vi "3D Model of Solar System.vi"() -> ()   [LabVIEW 2016]
doc: "This example demonstrates some fundamental concepts for the 3D picture. Concepts covered include object creation, texturing, object movement, and object hierarchy."
uses:
  <vilib>/Utility/miscctls.llb/LVRectTypeDef.ctl
  <vilib>/picture/3D Picture Control/Object/Create Object (drawable).vi
  <vilib>/picture/3D Picture Control/Helpers/Apply Texture (no reference).vi
  <vilib>/picture/3D Picture Control/Object/Create Object (name).vi
  <vilib>/picture/3D Picture Control/Object/Add Object (reference).vi
  <vilib>/picture/3D Picture Control/NI_3D Picture Control.lvlib
panel:
  in  "Rendering Destination":enum16{"Scene Window", "Scene Display"}(ring)=enum."Scene Display"
  in  "Camera Controller":enum16{"None", "Spherical", "Flying"}(ring)=enum."Spherical"
  out "Scene Display":refnum<vi>(3d-picture)
  in  "Stop":bool
  # "Overview: This example demonstrates some fundamental concepts for the 3D Picture by animating an image of the solar system.\nRequirements: LabVIEW Full Development System\nInstructions: \n1. Choose the Rendering Destination. If you choose Scene Window, a new window will show the rendering of the solar system. If you choose Scene Display, the picture will be shown in the Scene Display indicator on this front panel. \n2. Run the VI to see the animation of the solar system. \n3. Click Stop to stop the VI."
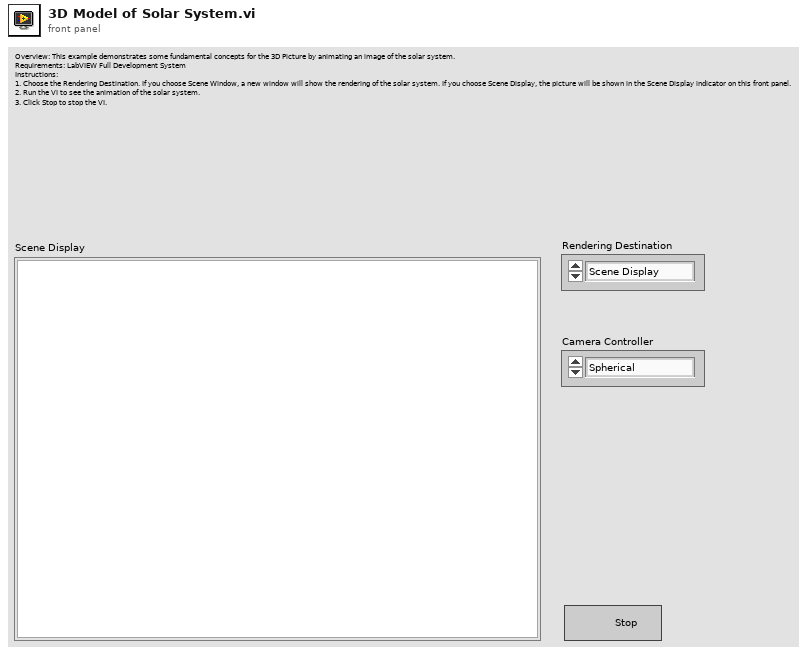
[diagram p1: front panel]
types:
  T1 = enum16{"As a Decal", "With Modulation", "With Blending", "As a replacement"}
  T2 = enum16{"No Filtration", "Linear Filtration", "Simple Mipmap Filtration", "Bilinear Filtration", "Trilinear Filtration"}
  T3 = typedef "imagedata.ctl" = cluster{"image type":i32, "image depth":i32, "image":u8[], "mask":u8[], "colors":u32[], "Rectangle":cluster{"left":i16, "top":i16, "right":i16, "bottom":i16}}
  T4 = enum16{"Open", "Minimized", "Maximized", "Hidden"}
  T5 = typedef "LVRectTypeDef.ctl" = cluster{"Left":i16, "Top":i16, "Right":i16, "Bottom":i16}
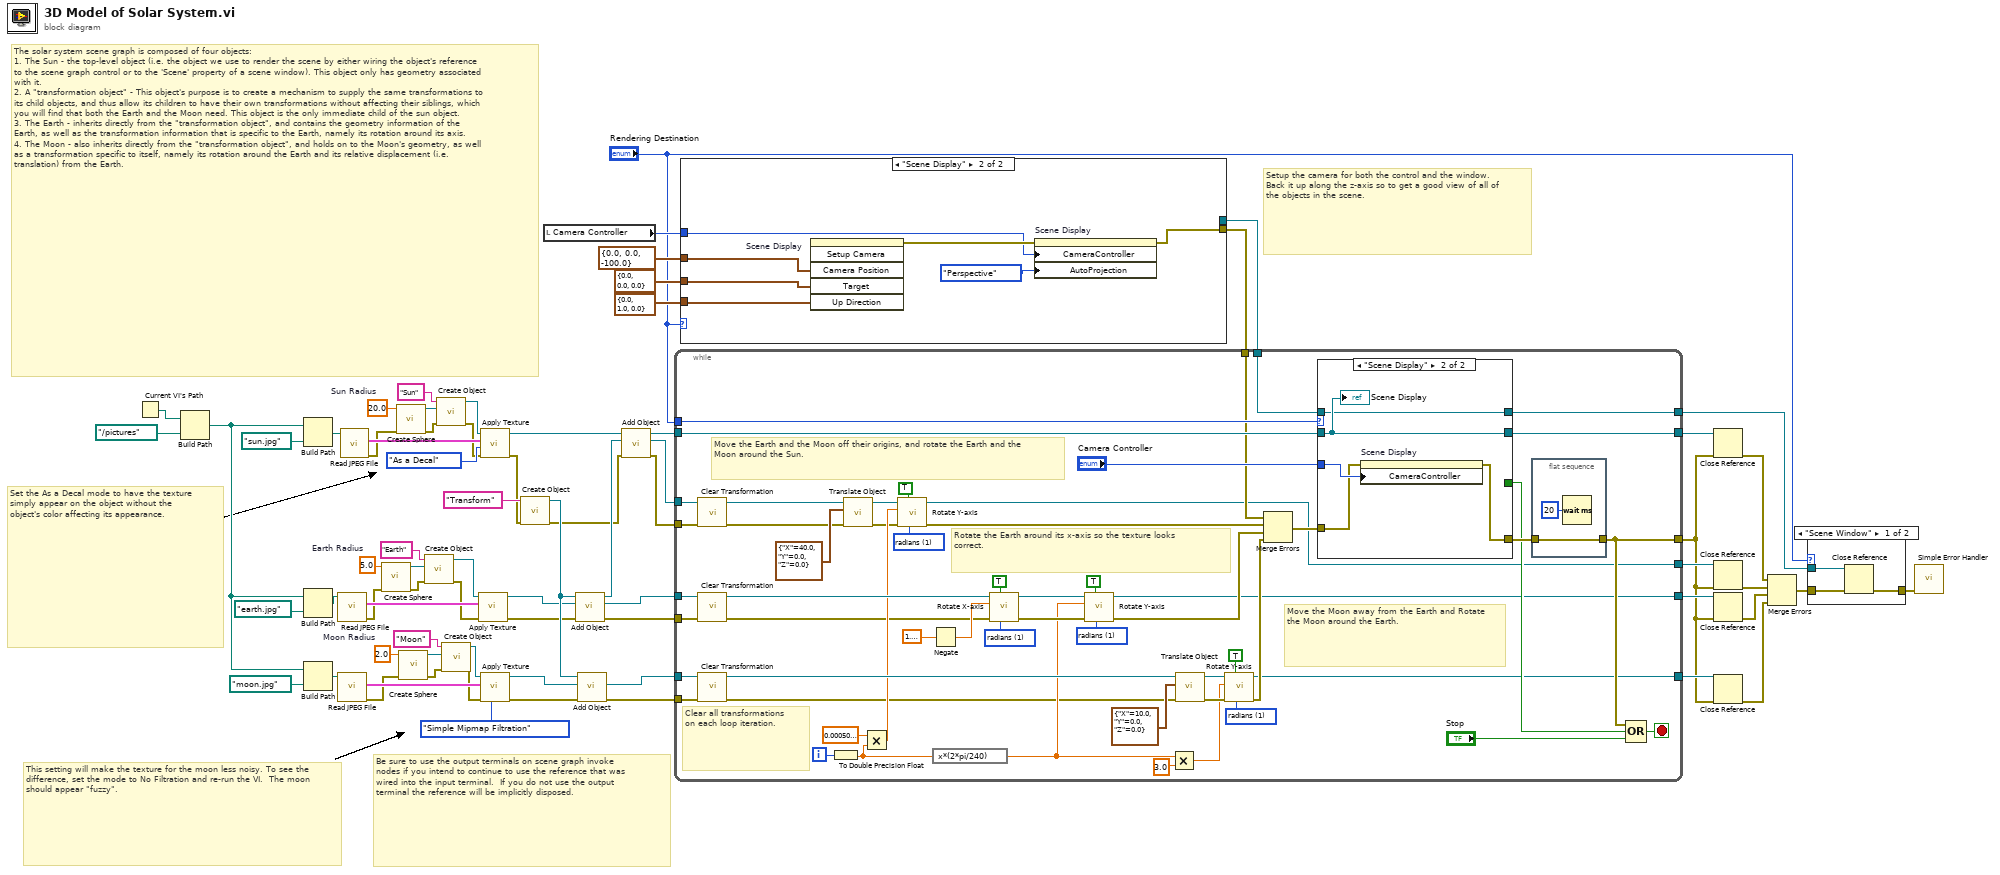
[diagram p0: block diagram]
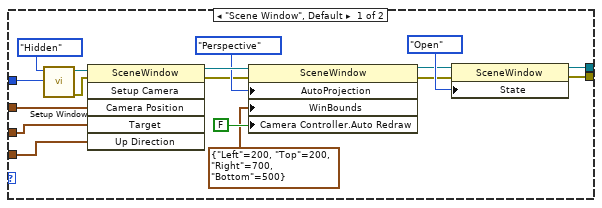
[diagram p3: hidden frame]
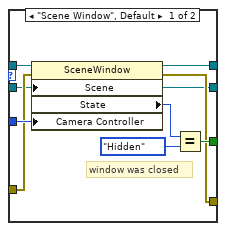
[diagram p4: hidden frame]
diagram:
  w68 = sgl 2.0  # Moon Radius
  w69 = sgl 5.0  # Earth Radius
  w70 = sgl 20.0  # Sun Radius
  # "Set the As a Decal mode to have the texture simply appear on the object without the object's color affecting its appearance."
  # "This setting will make the texture for the moon less noisy. To see the difference, set the mode to No Filtration and re-run the VI.  The moon should appear \"fuzzy\"."
  # "Be sure to use the output terminals on scene graph invoke nodes if you intend to continue to use the reference that was wired into the input terminal.  If you do not use the output terminal the reference will be implicitly disposed."
  # "Setup the camera for both the control and the window.  Back it up along the z-axis so to get a good view of all of the objects in the scene."
  # "The solar system scene graph is composed of four objects:\n1. The Sun - the top-level object (i.e. the object we use to render the scene by either wiring the object's reference to the scene graph control or to the 'Scene' property of a scene window). This object only has geometry associated with it.\n2. A \"transformation object\" - This object's purpose is to create a mechanism to supply the same transformations to its child objects, and thus allow its children to have their own transformations without affecting their siblings, which you will find that both the Earth and the Moon need. This object is the only immediate child of the sun object.\n3. The Earth - inherits directly from the \"transformation object\", and contains the geometry information of the Earth, as well as the transformation information that is specific to the Earth, namely its rotation around its axis.\n4. The Moon - also inherits directly from the \"transformation object\", and holds on to the Moon's geometry, as well as a transformation specific to itself, namely its rotation around the Earth and its relative displacement (i.e. translation) from the Earth."
  n1 = Current VI's Path() -> (path=w14:path)
  n2 = Build Path(base path=w14, name or relative path=path "../pictures" ("path")) -> (appended path=w17:path)
  n3 = Build Path(base path=w17, name or relative path=path "sun.jpg" ("Name")) -> (appended path=w66:path)
  n4 = Build Path(base path=w17, name or relative path=path "earth.jpg" ("Name")) -> (appended path=w64:path)
  n5 = Build Path(base path=w17, name or relative path=path "moon.jpg" ("Name")) -> (appended path=w62:path)
  n6 = call <vilib>:"Read JPEG File.vi"("path to JPEG file"=w64) -> ("error out"=w23:errorcluster, "image data"=w44:T3)  [unwired: 1 in, 8 out]
  n7 = call <vilib>:"Read JPEG File.vi"("path to JPEG file"=w62) -> ("error out"=w24:errorcluster, "image data"=w58:T3)  [unwired: 1 in, 8 out]
  n8 = call <vilib>:"Read JPEG File.vi"("path to JPEG file"=w66) -> ("error out"=w22:errorcluster, "image data"=w52:T3)  [unwired: 1 in, 8 out]
  n9 = call <vilib>:"Create Sphere.vi"("error in (no error)"=w23, "Radius"=w69) -> ("error out"=w26:errorcluster, "New Sphere Refnum"=w55:refnum<vi>)  [unwired: 1 in, 7 out]
  n10 = call <vilib>:"Create Sphere.vi"("error in (no error)"=w22, "Radius"=w70) -> ("error out"=w21:errorcluster, "New Sphere Refnum"=w42:refnum<vi>)  [unwired: 1 in, 7 out]
  n11 = call <vilib>:"Create Sphere.vi"("error in (no error)"=w24, "Radius"=w68) -> ("error out"=w28:errorcluster, "New Sphere Refnum"=w60:refnum<vi>)  [unwired: 1 in, 7 out]
  n12 = call-poly <vilib>:"Create Object.vi"("error in (no error)"=w26, "Geometry"=w55, "Name"="Earth") -> ("error out"=w25:errorcluster, "Scene:New Object"=w45:refnum<vi>)  [unwired: 7 in]
  n13 = call-poly <vilib>:"Create Object.vi"("error in (no error)"=w21, "Geometry"=w42, "Name"="Sun") -> ("error out"=w20:errorcluster, "Scene:New Object"=w53:refnum<vi>)  [unwired: 7 in]
  n14 = call-poly <vilib>:"Create Object.vi"("error in (no error)"=w28, "Geometry"=w60, "Name"="Moon") -> ("error out"=w27:errorcluster, "Scene:New Object"=w59:refnum<vi>)  [unwired: 7 in]
  n15 = call-poly <vilib>:"Apply Texture.vi"("error in (no error)"=w25, "Image Data"=w44, "Scene Object In"=w45) -> ("error out"=w34:errorcluster, "Scene Object Out"=w43:refnum<vi>)  [unwired: 7 in]
  n16 = call-poly <vilib>:"Apply Texture.vi"("error in (no error)"=w20, "Apply Mode"=T1."As a Decal", "Image Data"=w52, "Scene Object In"=w53) -> ("error out"=w19:errorcluster, "Scene Object Out"=w51:refnum<vi>)  [unwired: 6 in]
  n17 = call-poly <vilib>:"Apply Texture.vi"("Filter Mode"=T2."Simple Mipmap Filtration", "error in (no error)"=w27, "Image Data"=w58, "Scene Object In"=w59) -> ("error out"=w33:errorcluster, "Scene Object Out"=w57:refnum<vi>)  [unwired: 6 in]
  n18 = call-poly <vilib>:"Create Object.vi"("error in (no error)"=w19, "Name"="Transform") -> ("error out"=w32:errorcluster, "Scene:New Object"=w47:refnum<vi>)  [unwired: 8 in]
  n19 = local read "Camera Controller"() -> (w40:enum16{"None", "Spherical", "Flying"})
  n20 = call-poly <vilib>:"Add Object.vi"("error in (no error)"=w34, "New Object In"=w43, "Scene Object In"=w47) -> ("error out"=w30:errorcluster, "New Object Out"=w48:refnum<vi>, "Scene Object Out"=w46:refnum<vi>)  [unwired: 6 in]
  n21 = call-poly <vilib>:"Add Object.vi"("error in (no error)"=w33, "New Object In"=w57, "Scene Object In"=w47) -> ("error out"=w29:errorcluster, "New Object Out"=w18:refnum<vi>)  [unwired: 6 in, 1 out]
  n22 = call-poly <vilib>:"Add Object.vi"("error in (no error)"=w32, "New Object In"=w46, "Scene Object In"=w51) -> ("error out"=w31:errorcluster, "New Object Out"=w50:refnum<vi>, "Scene Object Out"=w49:refnum<vi>)  [unwired: 6 in]
  n23 = case shown="\"Scene Display\"" "Rendering Destination" {
    tunnel: w40 -> [w79 w93]
    tunnel: cluster{"X":sgl, "Y":sgl, "Z":sgl} {"X"=0.0, "Y"=0.0, "Z"=-100.0} ("Camera Position") -> [w81 w92]
    tunnel: cluster{"X":sgl, "Y":sgl, "Z":sgl} {"X"=0.0, "Y"=0.0, "Z"=0.0} ("Target") -> [w82 w91]
    tunnel: cluster{"X":sgl, "Y":sgl, "Z":sgl} {"X"=0.0, "Y"=1.0, "Z"=0.0} ("Up Direction") -> [w83 w90]
    tunnel: [w76 _] -> w36
    tunnel: [w72 w89] -> w15
    frame "Scene Window", Default {
      n24 = call <vilib>:"Setup Window.vi"("Camera Controller"=w79, "Window State"=T4."Hidden") -> ("error out"=w75:errorcluster, "New Window Refnum"=w85:refnum<vi>)  [unwired: 1 in, 7 out]
      n25 = invoke class="SceneWindow" method="Setup Camera"(reference=w85, error in=w75, "Camera Position"=w81, "Target"=w82, "Up Direction"=w83) -> (reference out=w84:refnum<vi>, error out=w74:errorcluster)  [unwired: 1 in, 4 out]
      n26 = property class="SceneWindow"(reference=w84, error in=w74, "AutoProjection"=enum16{"None", "Perspective", "Orthographic"}."Perspective" ("Automatic Projection Mode"), "WinBounds"=T5 {"Left"=200, "Top"=200, "Right"=700, "Bottom"=500} ("Window Bounds"), "Camera Controller.Auto Redraw"=FALSE ("Camera Controller:Auto Redraw")) -> (reference out=w77:refnum<vi>, error out=w73:errorcluster)
      n27 = property class="SceneWindow"(reference=w77, error in=w73, "State"=T4."Open" ("Window State")) -> (reference out=w76:refnum<vi>, error out=w72:errorcluster)
    }
    frame "Scene Display" {
      n28 = invoke on="Scene Display" class="SceneGraphDisp (strict)" method="Setup Camera"("Camera Position"=w92, "Target"=w91, "Up Direction"=w90) -> (error out=w94:errorcluster)  [unwired: 3 in, 5 out]
      n29 = property on="Scene Display" class="SceneGraphDisp (strict)"(error in=w94, "CameraController"=w93, "AutoProjection"=enum16{"None", "Perspective", "Orthographic"}."Perspective" ("Auto Projection Mode")) -> (error out=w89:errorcluster)  [unwired: 1 in, 1 out]
    }
  }
  n30 = while {
    tunnel: w36 -> [w149]
    tunnel: w49 -> [w148]
    tunnel: w50 -> [w147]
    tunnel: w48 -> [w146]
    tunnel: w18 -> [w145]
    tunnel: "Rendering Destination" -> [w144]
    tunnel: w31 -> [w115]
    tunnel: w30 -> [w113]
    tunnel: w29 -> [w112]
    tunnel: [w110] -> w4
    tunnel: w15 -> [w103]
    tunnel: [w100] -> w13
    tunnel: [w99] -> w11
    tunnel: [w98] -> w12
    tunnel: [w97] -> w10
    tunnel: [w96] -> w5
    i -> [w151]
    stop <- w111 stop-if-true
    w124 = u16 1 items=["degree", "radians"] ("angle unit")
    w125 = u16 1 items=["degree", "radians"] ("angle unit")
    w126 = u16 1 items=["degree", "radians"] ("angle unit")
    w127 = u16 1 items=["degree", "radians"] ("angle unit")
    # "Move the Moon away from the Earth and Rotate the Moon around the Earth."
    # "Rotate the Earth around its x-axis so the texture looks correct."
    # "Move the Earth and the Moon off their origins, and rotate the Earth and the Moon around the Sun."
    # "Clear all transformations on each loop iteration."
    n31 = call <vilib>:"Clear Transformation.vi"("error in (no error)"=w115, "Object Refnum In"=w147) -> ("error out"=w114:errorcluster, "Object Refnum Out"=w143:refnum<vi>)  [unwired: 8 out]
    n32 = call <vilib>:"Clear Transformation.vi"("error in (no error)"=w113, "Object Refnum In"=w146) -> ("error out"=w109:errorcluster, "Object Refnum Out"=w142:refnum<vi>)  [unwired: 8 out]
    n33 = call <vilib>:"Clear Transformation.vi"("error in (no error)"=w112, "Object Refnum In"=w145) -> ("error out"=w108:errorcluster, "Object Refnum Out"=w141:refnum<vi>)  [unwired: 8 out]
    n34 = To Double Precision Float(number=w151) -> (double precision float=w150:dbl)
    n35 = call <vilib>:"Translate Object.vi"("error in (no error)"=w114, "Translation"=cluster{"X":sgl, "Y":sgl, "Z":sgl} {"X"=40.0, "Y"=0.0, "Z"=0.0}, "Scene.Object In"=w143) -> ("error out"=w135:errorcluster, "Scene.Object Out"=w136:refnum<vi>)  [unwired: 7 out]
    n36 = Multiply(x=sgl 0.0005 ("Angle"), y=w150) -> (x*y=w139:dbl)
    n37 = call <vilib>:"Rotate Y-axis.vi"("angle unit"=w124, "Relative?"=TRUE, "error in (no error)"=w135, "angle"=w139, "Scene Object In"=w136) -> ("error out"=w107:errorcluster, "Scene Object Out"=w97:refnum<vi>)  [unwired: 5 in]
    n38 = Negate(x=1.5707963267948966) -> (-x=w130:dbl)
    n39 = expression code="x*(2*pi/240)"(w150) -> (w119:dbl)
    n40 = call <vilib>:"Rotate X-axis.vi"("angle unit"=w127, "Relative?"=TRUE, "error in (no error)"=w109, "angle"=w130, "Scene Object In"=w142) -> ("error out"=w132:errorcluster, "Scene Object Out"=w133:refnum<vi>)  [unwired: 5 in]
    n41 = call <vilib>:"Rotate Y-axis.vi"("angle unit"=w126, "Relative?"=TRUE, "error in (no error)"=w132, "angle"=w119, "Scene Object In"=w133) -> ("error out"=w106:errorcluster, "Scene Object Out"=w98:refnum<vi>)  [unwired: 5 in]
    n42 = Multiply(x=w119, y=3.0) -> (x*y=w128:dbl)
    n43 = call <vilib>:"Translate Object.vi"("error in (no error)"=w108, "Translation"=cluster{"X":sgl, "Y":sgl, "Z":sgl} {"X"=10.0, "Y"=0.0, "Z"=0.0}, "Scene.Object In"=w141) -> ("error out"=w134:errorcluster, "Scene.Object Out"=w137:refnum<vi>)  [unwired: 7 out]
    n44 = call <vilib>:"Rotate Y-axis.vi"("angle unit"=w125, "Relative?"=TRUE, "error in (no error)"=w134, "angle"=w128, "Scene Object In"=w137) -> ("error out"=w105:errorcluster, "Scene Object Out"=w99:refnum<vi>)  [unwired: 5 in]
    n45 = Merge Errors(w103, w107, w106, w105) -> (w104:errorcluster)
    n46 = case shown="\"Scene Display\"" w144 {
      tunnel: w149 -> [w162 w163]
      tunnel: w148 -> [w155 w164]
      tunnel: w104 -> [w157 w166]
      tunnel: [w156 w165] -> w117
      tunnel: [w159 _] -> w101
      tunnel: "Camera Controller" -> [w158 w167]
      tunnel: [w155 w164] -> w100
      tunnel: [w154 w163] -> w96
      frame "Scene Window", Default {
        # "window was closed"
        n47 = property class="SceneWindow"(reference=w162, error in=w157, "Scene"=w155, "Camera Controller"=w158) -> (reference out=w154:refnum<vi>, error out=w156:errorcluster, "State"=w161:T4)
        n48 = Equal?(x=w161, y=T4."Hidden" ("Window State")) -> (x = y?=w159:bool)
      }
      frame "Scene Display" {
        n49 = property on="Scene Display" class="SceneGraphDisp (strict)"(error in=w166, "CameraController"=w167) -> (error out=w165:errorcluster)  [unwired: 1 in, 1 out]
        "Scene Display" <- w164
      }
    }
    n50 = flat-sequence {
      tunnel: w117 -> [w153]
      tunnel: [w153] -> w110
      frame #0 {
        n51 = Wait (ms)(milliseconds to wait=u32 20) -> ()  [unwired: 1 out]
      }
    }
    n52 = Compound Arithmetic op=OR(w110, w101, "Stop") -> (w111:bool)
  }
  n53 = Close Reference(reference=w13, error in (no error)=w4) -> (error out=w9:errorcluster)
  n54 = Close Reference(reference=w10, error in (no error)=w4) -> (error out=w8:errorcluster)
  n55 = Close Reference(reference=w12, error in (no error)=w4) -> (error out=w7:errorcluster)
  n56 = Close Reference(reference=w11, error in (no error)=w4) -> (error out=w6:errorcluster)
  n57 = Merge Errors(w9, w8, w7, w6) -> (w3:errorcluster)
  n58 = case shown="\"Scene Window\"" "Rendering Destination" {
    tunnel: w5 -> [w170 _]
    tunnel: w3 -> [w169 w171]
    tunnel: [w168 w171] -> w2
    frame "Scene Window" {
      n59 = Close Reference(reference=w170, error in (no error)=w169) -> (error out=w168:errorcluster)
    }
    frame "Scene Display", Default {
    }
  }
  n60 = call <vilib>:"Simple Error Handler.vi"("error in (no error)"=w2) -> ()  [unwired: 4 in, 5 out]
